vi "Create Play.vi"(0 "Filename Array in":string[](array[string]), 2 "Empty Play Definition":T1, 5 "Application Directory":path, 7 "Play Selection Box Property Reference":refnum<vi>, 9 "Create New Play":bool, 11 "Filepath Array in":string[](array[string])) -> (4 "Load New Play":bool, 6 "Filepath Array out":string[](array[string]), 10 "Filename Array out":string[](array[string]), 15 "error out":errorcluster)   [LabVIEW 2016]
uses:
  Autonomous VIs/Autonomous Exec/Autonomous Play Definition.ctl
  Autonomous VIs/Autonomous Commands/Autonomous Command Names.ctl
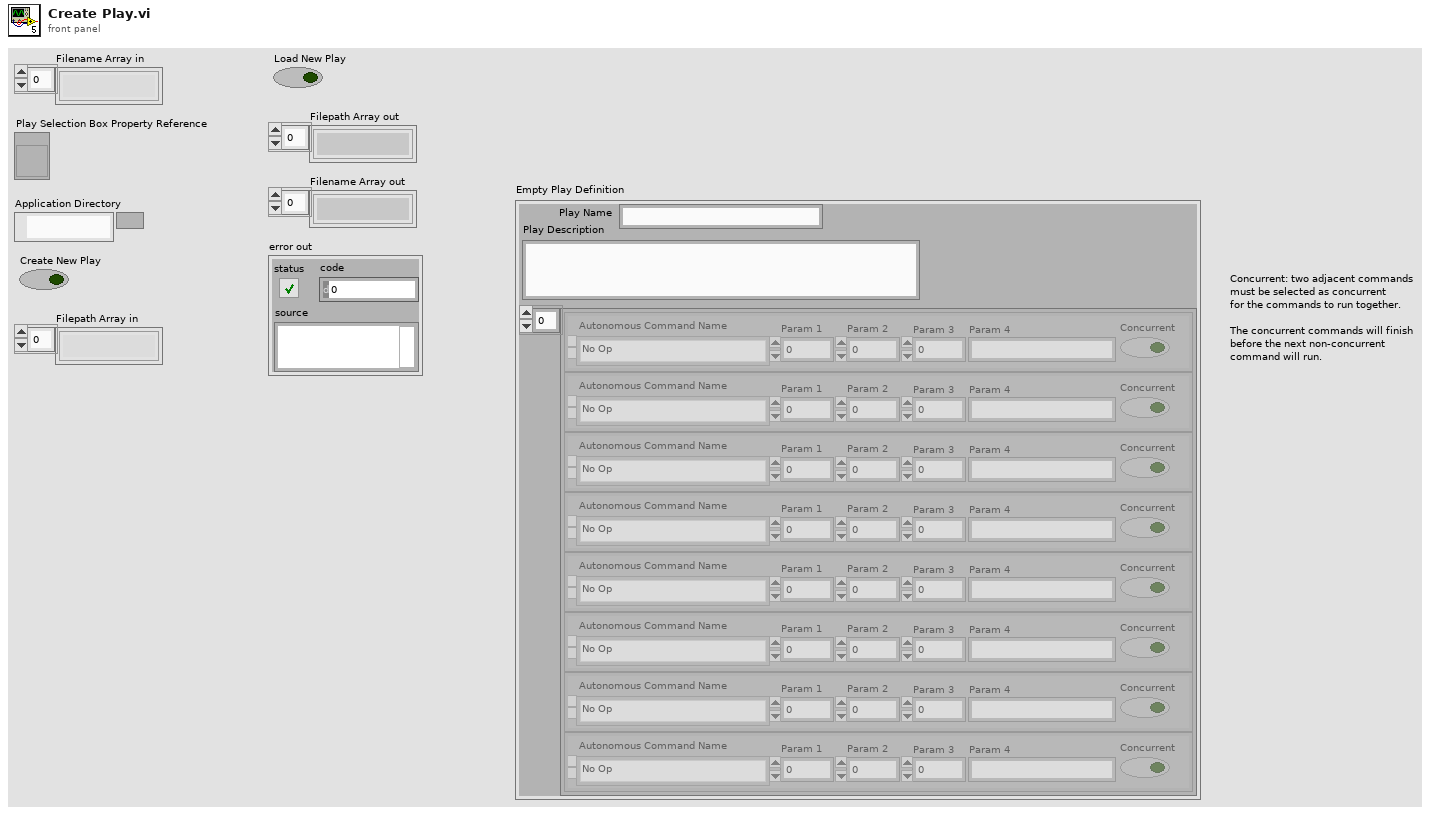
[diagram p1: front panel]
types:
  T1 = typedef "Autonomous Play Definition.ctl" = cluster{"Play Name":string, "Command List":cluster{"Param 1":dbl, "Param 2":dbl, "Autonomous Command Name":T2, "Concurrent":bool, "Param 3":dbl, "Param 4":string}[], "Play Description":string}
  T2 = typedef "Autonomous Command Names.ctl" = enum16{"No Op", "Command Drive+Climb Shift", "Command Wait", "Command Deliver Gear", "Command Buffer", "Command Drive Path"}
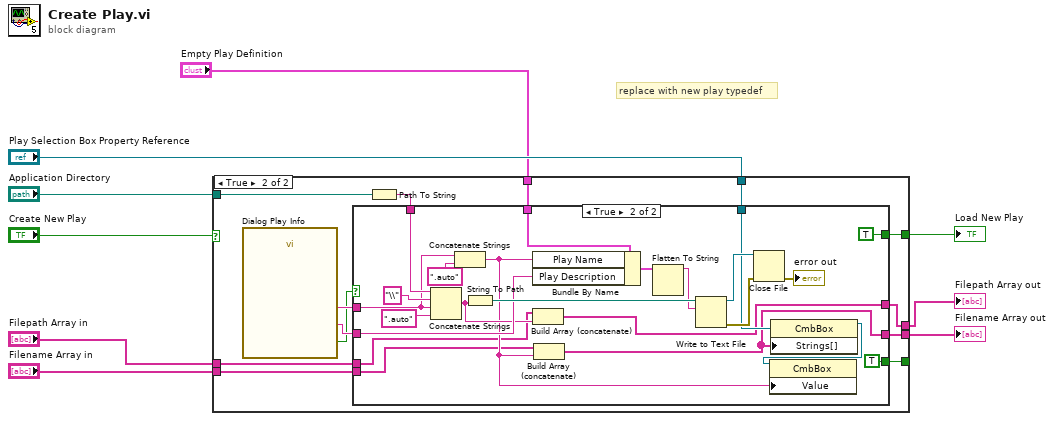
[diagram p0: block diagram]
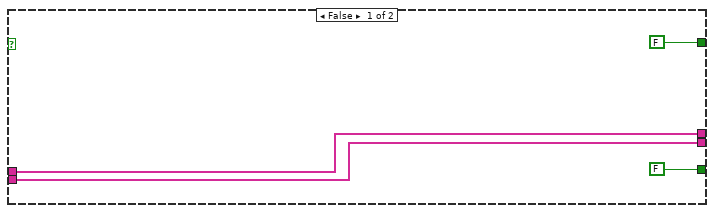
[diagram p2: hidden frame]
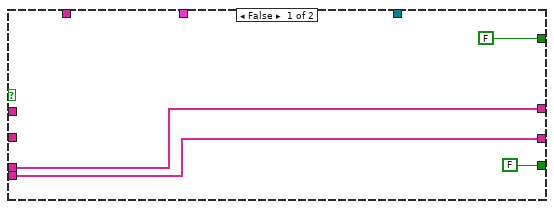
[diagram p3: hidden frame]
diagram:
  # "replace with new play typedef"
  n1 = case shown="True" "Create New Play" {
    tunnel: [FALSE ("value") w22] -> _
    tunnel: [FALSE w21] -> w3
    tunnel: "Application Directory" -> [_ w20]
    tunnel: "Play Selection Box Property Reference" -> [_ w19]
    tunnel: "Filepath Array in" -> [w11 w18]
    tunnel: "Filename Array in" -> [w10 w17]
    tunnel: [w11 w16] -> w8
    tunnel: [w10 w15] -> w9
    tunnel: "Empty Play Definition" -> [_ w14]
    frame False {
    }
    frame True {
      n2 = call "Dialog Play Info.vi"() -> ("Play Description ind"=w25:string, "Play Name ind"=w24:string, "OK ind"=w23:bool)  [unwired: 16 in, 1 out]
      n3 = Path To String(path=w20) -> (string=w26:string)
      n4 = case shown="True" w23 {
        tunnel: w26 -> [_ w52]
        tunnel: w25 -> [_ w49]
        tunnel: w24 -> [_ w42]
        tunnel: [FALSE ("value") TRUE ("value")] -> w22
        tunnel: [FALSE TRUE] -> w21
        tunnel: w19 -> [_ w36]
        tunnel: w18 -> [w28 w35]
        tunnel: w17 -> [w27 w34]
        tunnel: [w28 w33] -> w16
        tunnel: [w27 w32] -> w15
        tunnel: w14 -> [_ w31]
        frame False {
        }
        frame True {
          n5 = Concatenate Strings(w52, "\\" ("string"), w42, ".auto" ("string")) -> (w43:string)
          n6 = Concatenate Strings(w42, ".auto" ("string")) -> (w40:string)
          n7 = String To Path(string=w43) -> (path=w50:path)
          n8 = Bundle By Name(cluster=w31, "Play Name"=w40, "Play Description"=w49) -> (w48:T1)
          n9 = Build Array (concatenate)(w35, w43) -> (w33:string[])
          n10 = Build Array (concatenate)(w34, w40) -> (w32:string[])
          n11 = Flatten To String(anything=w48) -> (data string=w47:string)  [unwired: 3 in, 2 out]
          n12 = Write to Text File(file (use dialog)=w50, text=w47) -> (refnum out=w39:refnum<file>, error out=w38:errorcluster)  [unwired: 2 in, 1 out]
          n13 = Close File(refnum=w39, error in=w38) -> (error out=→"error out":errorcluster)  [unwired: 1 out]
          n14 = property class="CmbBox"(reference=w36, "Strings[]"=w32) -> (reference out=w44:refnum<vi>)  [unwired: 1 in, 1 out]
          n15 = property class="CmbBox"(reference=w44, "Value"=w40) -> ()  [unwired: 1 in, 2 out]
        }
      }
    }
  }
  "Filename Array out" <- w9
  "Filepath Array out" <- w8
  "Load New Play" <- w3
